vi "test.vi"(8 "COLUMN":i32=9, 9 "ROW":i32=6, 10 "引用":refnum<vi>) -> (0 "料盘ID NG？":bool, 1 "条码1":string[][](array[string]), 2 "条码字符串":string, 3 "托盘ID":string, 4 "工位一NG?":bool, 5 "46~99条码数组":string[](array[string]), 6 "工位1逻辑与":bool)   [LabVIEW 2014]
uses:
  <vilib>/Utility/miscctls.llb/LVRowAndColumnTypeDef.ctl
panel:
  out "已删除的部分 2":string[](array[string])
  out "已删除元素的数组子集 2":string[](array[string])
  out "元素索引 2":i32
  out "数组 3":string[](array[string])
  out "初始化的数组":u32[][](array[numeric])
  out "数组 2":u32[][](array[numeric])
  out "颜色数组":u32[][](array[numeric])
  in  "多列列表框 2":i32[](listbox)
  out "条码数组":string[](array[string])
  out "大小":i32
  out "x-y":dbl
  out "工位1表格":string[][](array[string])
  # "16777238"
  # "Infomation"
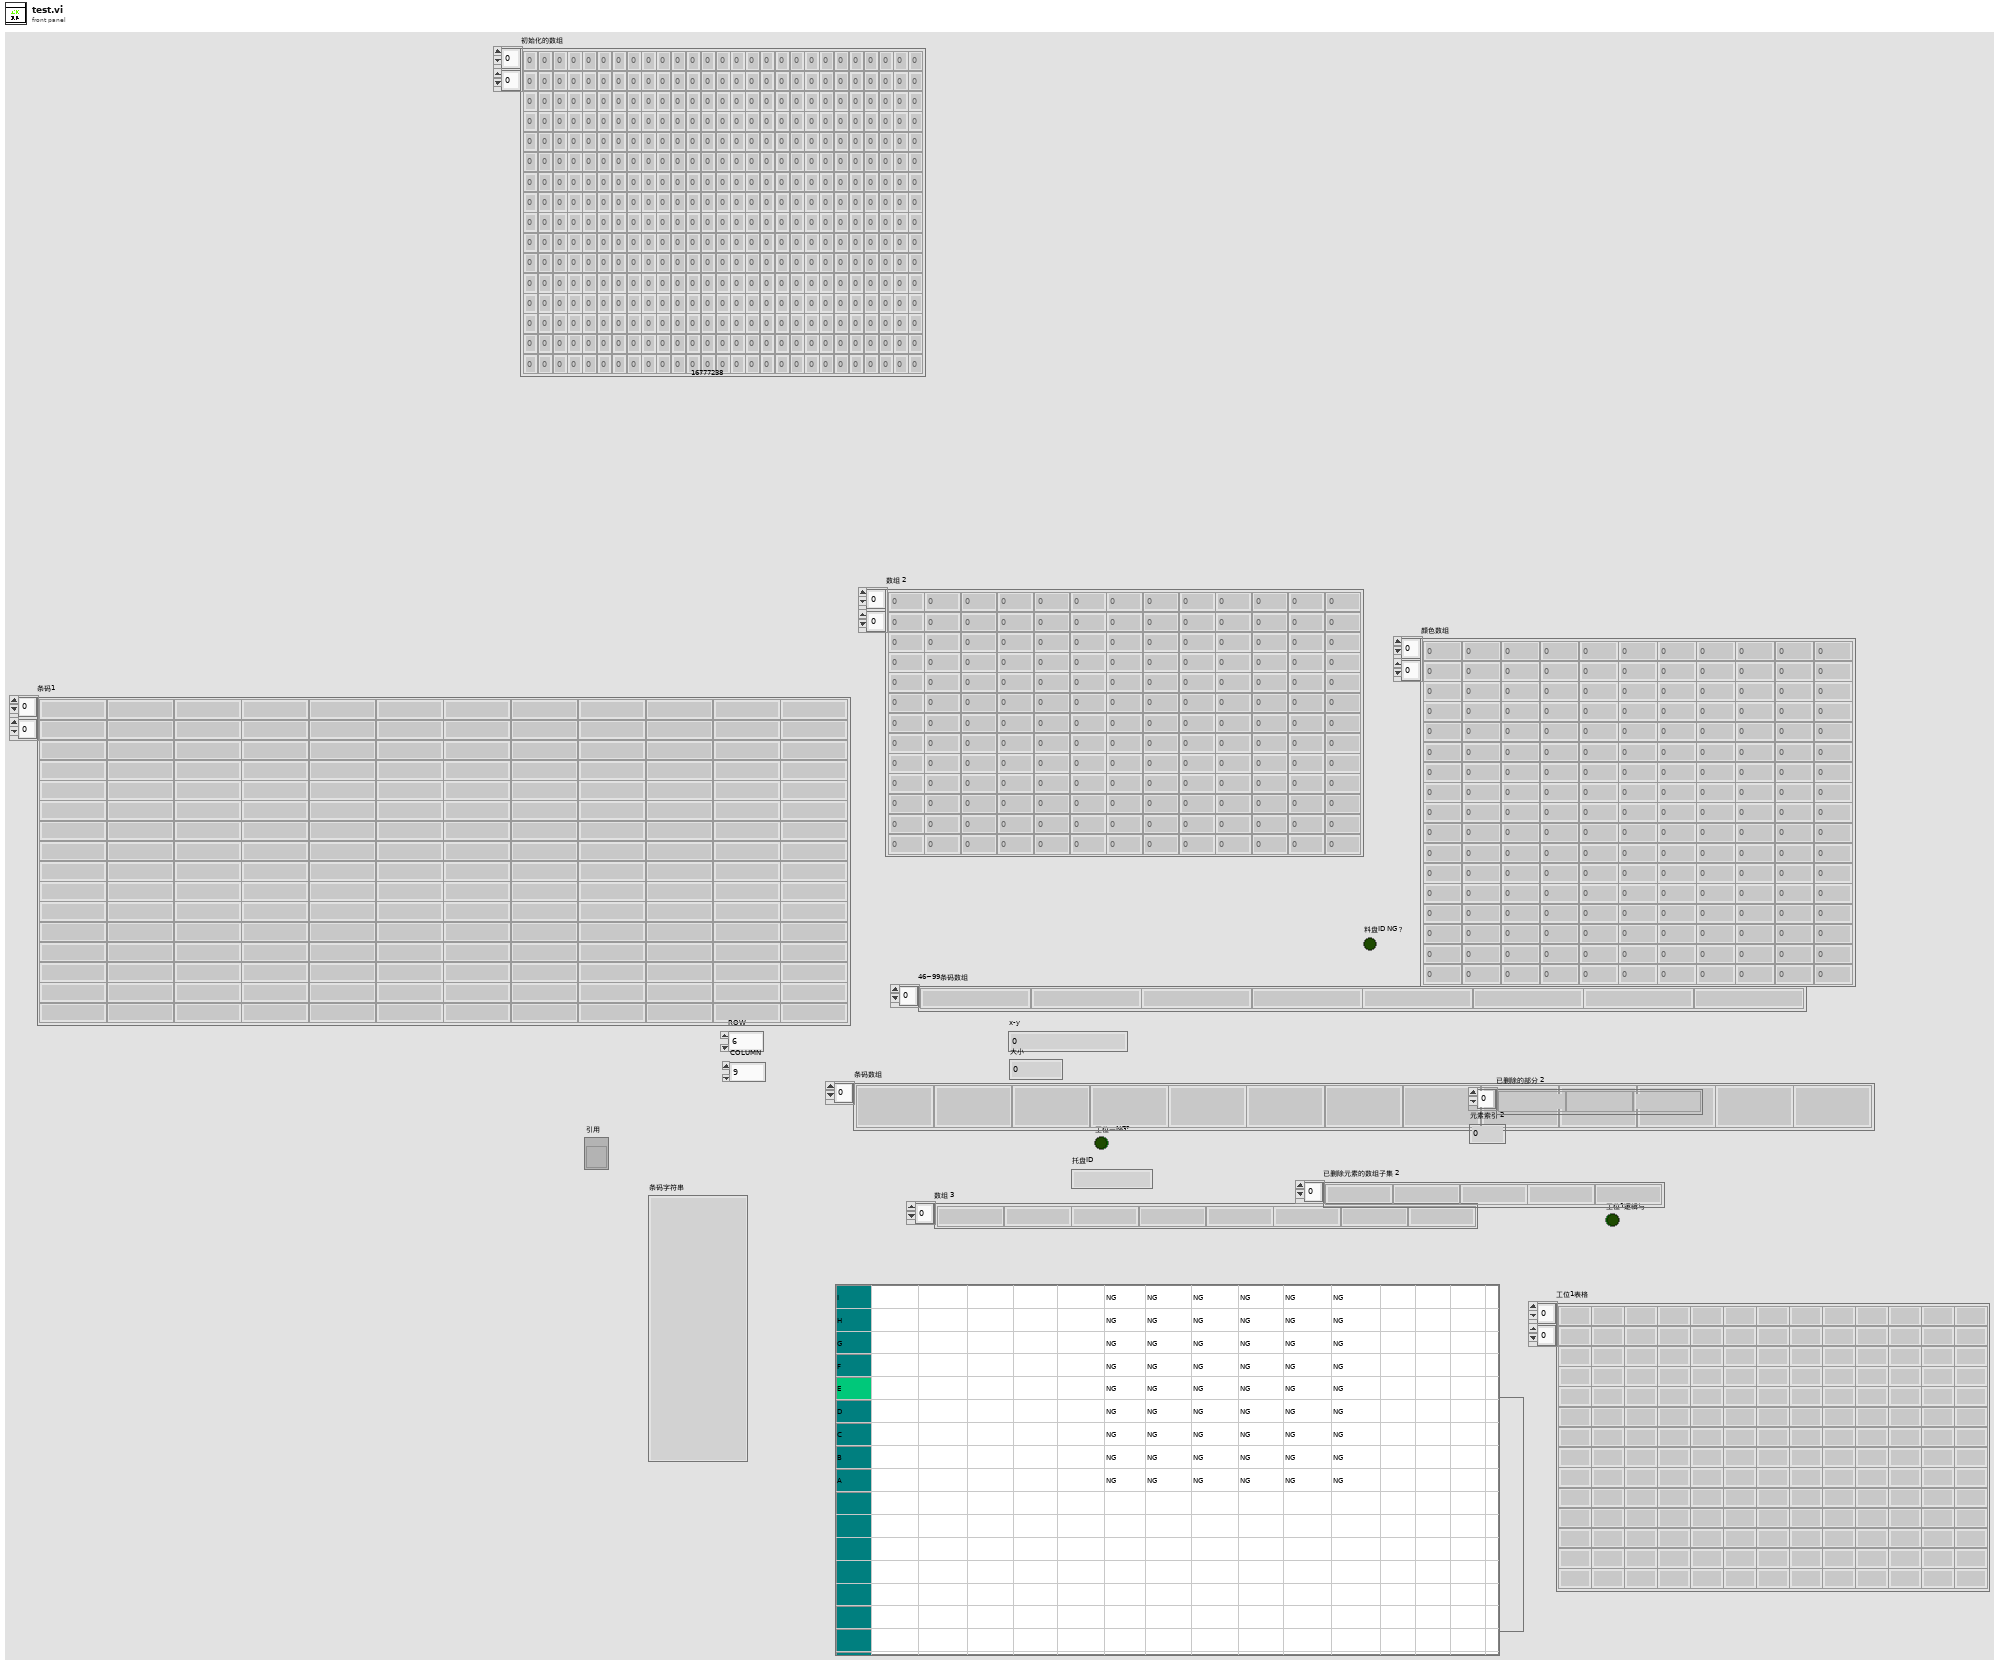
[diagram p1: front panel]
types:
  T1 = typedef "LVRowAndColumnTypeDef.ctl" = cluster{"Row":i32, "Column":i32}
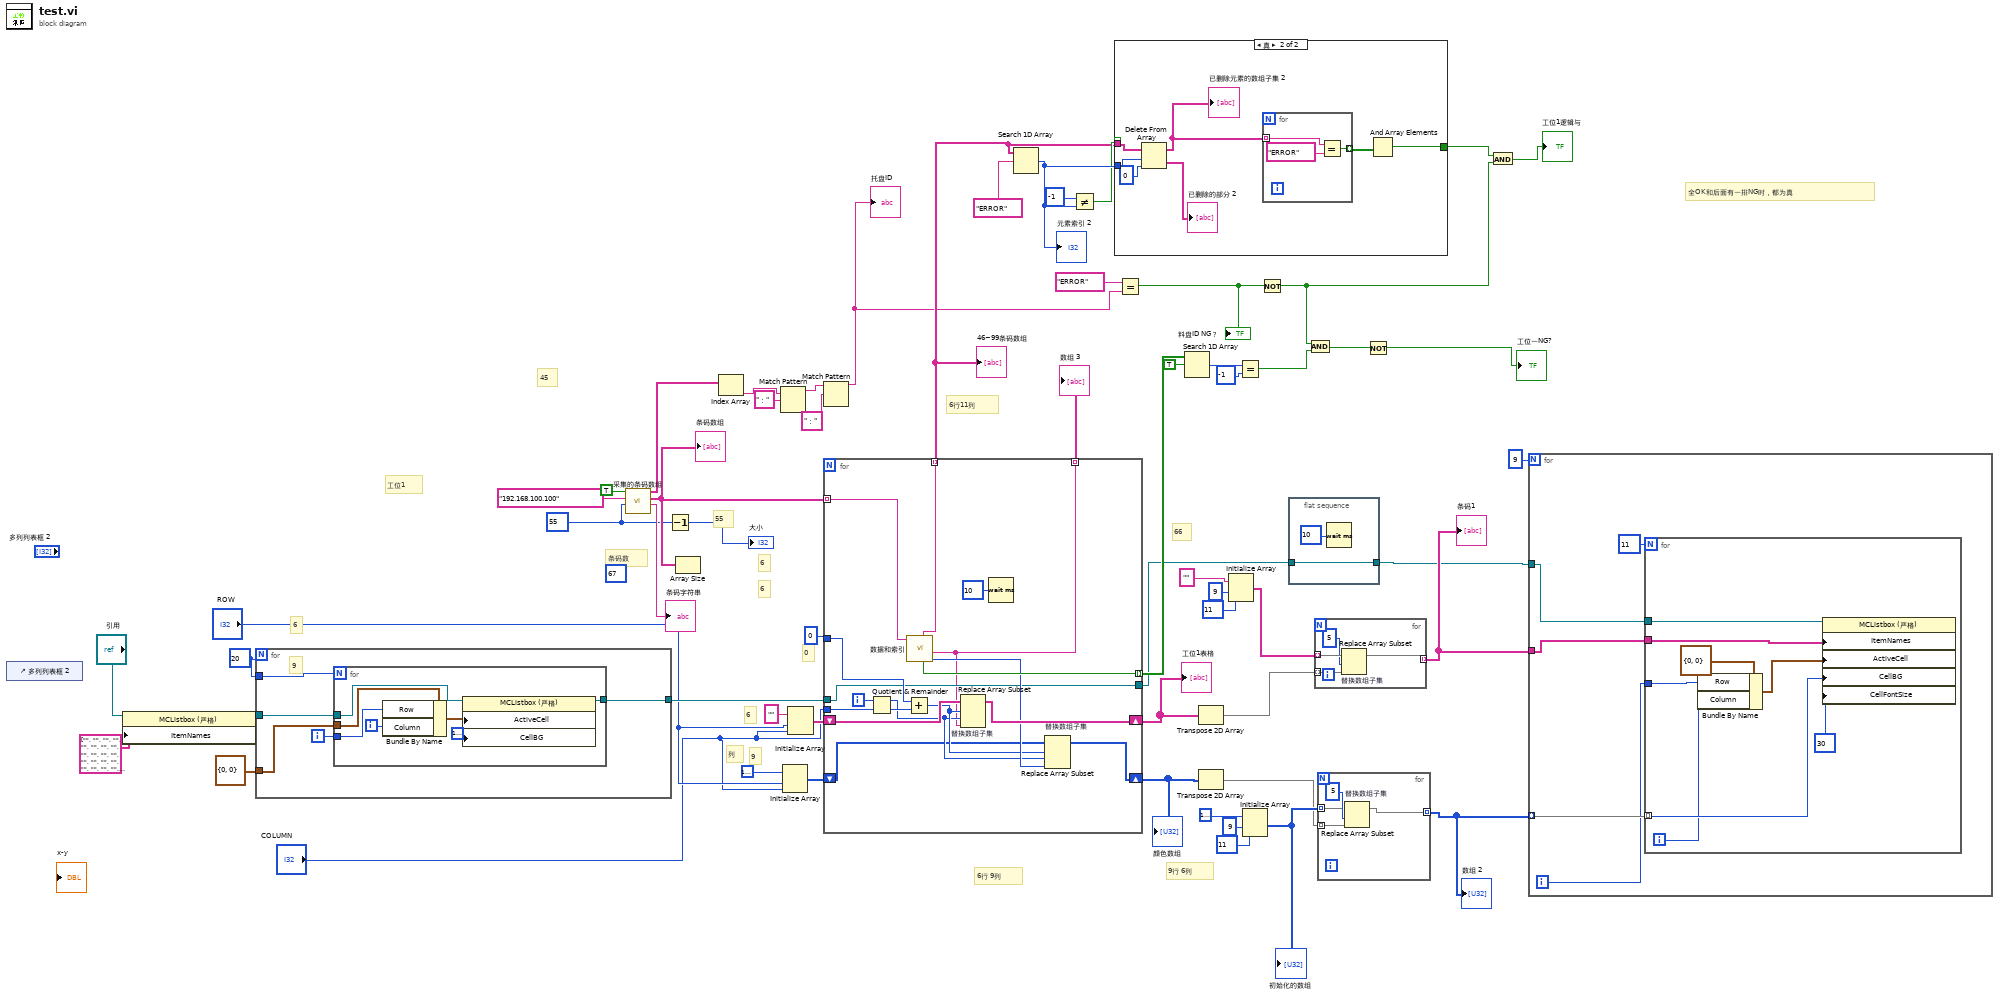
[diagram p0: block diagram]
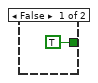
[diagram p2: hidden frame]
diagram:
  w23 = 20
  (unwired) 67
  w46 = 55 ("条码数量")
  # "全OK和后面有一排NG时，都为真"
  # "工位1"
  # "45"
  # "9行 6列"
  # "6行 9列"
  # "66"
  # "6"
  # "6"
  # "6行11列"
  # "0"
  # "条码数"
  # "6"
  # "6"
  # "55"
  # "9"
  # "列"
  n1 = control-ref of="多列列表框 2"() -> ()  [unwired: 1 out]
  n2 = property class="MCListbox (严格)"(reference="引用", "ItemNames"=string[][] [["", "", "", "", "", "", "", "", "", "", ""], ["", "", "", "", "", "", "", "", "", "", ""], ["", "", "", "", "", "", "", "", "", "", ""], ["", "", "", "", "", "", "", "", "", "", ""], ["", "", "", "", "", "", "", "", "", "", ""]] ("项名")) -> (reference out=w58:refnum<vi>)  [unwired: 1 in, 1 out]
  n3 = for {
    N: w23 -> [_]
    tunnel: w58 -> [w65]
    tunnel: T1 {"Row"=0, "Column"=0} ("活动单元格:活动单元格") -> [w64]
    tunnel: [w62] -> w57
    tunnel: w23 -> [w61]
    i -> [w63]
    # "9"
    n4 = for {
      N: w61 -> [_]
      tunnel: w65 -> [w72]
      tunnel: w64 -> [w71]
      tunnel: w63 -> [w69]
      tunnel: [w67] -> w62
      i -> [w68]
      n5 = Bundle By Name(cluster=w71, "Row"=w69, "Column"=w68) -> (w70:T1)
      n6 = property class="MCListbox (严格)"(reference=w72, "ActiveCell"=w70, "CellBG"=u32 16777238) -> (reference out=w67:refnum<vi>)  [unwired: 1 in, 1 out]
    }
  }
  n7 = call "采集的条码数组.vi"("条码数量"=w46, "地址"="192.168.100.100", "开启条码?"=TRUE) -> ("条码字符串"=→"条码字符串":string, "条码数组"=w47:string[], "料号"=w20:string[])  [unwired: 6 in]
  "条码数组" <- w47
  n8 = Decrement(x=w46) -> (x-1=→"大小":i32)
  n9 = Array Size(array=w47) -> ()  [unwired: 1 out]
  n10 = Index Array(array=w20) -> (element=w19:string)  [unwired: 1 in]
  n11 = Match Pattern(string=w19, regular expression="：" ("正则表达式")) -> (before substring=w17:string)  [unwired: 1 in, 3 out]
  n12 = Initialize Array(u32 16777238, "ROW", "COLUMN") -> (w43:u32[][])
  n13 = Initialize Array("", "ROW", "COLUMN") -> (w48:string[][])
  n14 = Match Pattern(string=w17, regular expression="：" ("正则表达式")) -> (before substring=w8:string)  [unwired: 1 in, 3 out]
  "托盘ID" <- w8
  n15 = for {
    tunnel: w47 -> [w89] mode=indexing
    tunnel: w57 -> [w76]
    shift-right: [w88] -> w42
    shift-left: w48 -> [w82]
    tunnel: [w87] -> w56 mode=indexing
    tunnel: "COLUMN" -> [w85]
    tunnel: 0 -> [w83]
    shift-right: [w77] -> w41
    shift-left: w43 -> [w78]
    tunnel: [w76] -> w30
    tunnel: [w74] -> w22 mode=indexing
    tunnel: [w73] -> w10 mode=indexing
    i -> [w86]
    n16 = Quotient & Remainder(x=w86, y=w85) -> (x-y*floor(x/y)=w79:i32, floor(x/y)=w84:i32)
    n17 = Add(x=w83, y=w84) -> (x+y=w80:i32)
    n18 = call "数据和索引.vi"("data out"=w89) -> ("颜色"=w81:u32, "显示数据"=w74:string, "NG?"=w87:bool, "条码"=w73:string)  [unwired: 6 in, 1 out]
    n19 = Replace Array Subset "替换数组子集"(array=w82, new element=w74, index (row)=w80, index (col)=w79) -> (w88:string[][])
    n20 = Wait (ms)(milliseconds to wait=u32 10 ("等待时间（毫秒）")) -> ()  [unwired: 1 out]
    n21 = Replace Array Subset "替换数组子集"(array=w78, new element=w81, index (row)=w80, index (col)=w79) -> (w77:u32[][])
  }
  "工位1表格" <- w42
  "颜色数组" <- w41
  "数组 3" <- w22
  "46~99条码数组" <- w10
  n22 = Search 1D Array(1D array=w10, element="ERROR") -> (index of element=w13:i32)  [unwired: 1 in]
  "元素索引 2" <- w13
  n23 = Not Equal?(x=-1, y=w13) -> (x != y?=w12:bool)
  n24 = case shown="真" w12 {
    tunnel: [TRUE w97] -> w6
    tunnel: w10 -> [_ w96]
    tunnel: w13 -> [_ w95]
    frame False {
    }
    frame True {
      n25 = Delete From Array(array=w96, length=w95, index=0 ("索引")) -> (deleted portion=→"已删除的部分 2":string[], array with subset deleted=w92:string[])
      "已删除元素的数组子集 2" <- w92
      n26 = for {
        tunnel: w92 -> [w100] mode=indexing
        tunnel: [w98] -> w91 mode=indexing
        n27 = Equal?(x=w100, y="ERROR") -> (x = y?=w98:bool)
      }
      n28 = And Array Elements(Boolean array=w91) -> (logical AND=w97:bool)
    }
  }
  n29 = Equal?(x="ERROR", y=w8) -> (x = y?=w7:bool)
  "料盘ID NG？" <- w7
  n30 = Search 1D Array(1D array=w56, element=TRUE) -> (index of element=w54:i32)  [unwired: 1 in]
  n31 = Transpose 2D Array(2D array=w42) -> (transposed array=w35:string[][])
  n32 = Transpose 2D Array(2D array=w41) -> (transposed array=w25:u32[][])
  n33 = Initialize Array("", 9 ("维数大小"), 11 ("维数大小")) -> (w36:string[][])
  n34 = Equal?(x=w54, y=-1) -> (x = y?=w4:bool)
  n35 = Initialize Array(u32 16777238, 9 ("维数大小"), 11 ("维数大小")) -> (w26:u32[][])
  "初始化的数组" <- w26
  n36 = Not(x=w7) -> (.not. x?=w3:bool)
  n37 = flat-sequence {
    tunnel: w30 -> [w102]
    tunnel: [w102] -> w29
    frame #0 {
      n38 = Wait (ms)(milliseconds to wait=u32 10 ("等待时间（毫秒）")) -> ()  [unwired: 1 out]
    }
  }
  n39 = And(x=w3, y=w4) -> (x .and. y?=w2:bool)
  n40 = for {
    tunnel: w36 -> [w106] mode=indexing
    tunnel: w35 -> [w105] mode=indexing
    tunnel: [w103] -> w31 mode=indexing
    n41 = Replace Array Subset "替换数组子集"(array=w106, new element=w105, index=5 ("索引")) -> (w103:string[])
  }
  "条码1" <- w31
  n42 = for {
    tunnel: w26 -> [w107] mode=indexing
    tunnel: w25 -> [w110] mode=indexing
    tunnel: [w108] -> w27 mode=indexing
    n43 = Replace Array Subset "替换数组子集"(array=w107, new element=w110, index=5 ("索引")) -> (w108:u32[])
  }
  "数组 2" <- w27
  n44 = Not(x=w2) -> (.not. x?=→"工位一NG?":bool)
  n45 = And(x=w6, y=w3) -> (x .and. y?=→"工位1逻辑与":bool)
  n46 = for {
    N: 9 -> [_]
    tunnel: w31 -> [w115]
    tunnel: w29 -> [w114]
    tunnel: w27 -> [w113] mode=indexing
    i -> [w111]
    n47 = for {
      N: 11 -> [_]
      tunnel: w115 -> [w123]
      tunnel: w114 -> [w122]
      tunnel: w113 -> [w118] mode=indexing
      tunnel: w111 -> [w117]
      i -> [w116]
      n48 = Bundle By Name(cluster=T1 {"Row"=0, "Column"=0} ("活动单元格:活动单元格"), "Row"=w117, "Column"=w116) -> (w120:T1)
      n49 = property class="MCListbox (严格)"(reference=w122, "ItemNames"=w123, "ActiveCell"=w120, "CellBG"=w118, "CellFontSize"=u32 30 ("活动单元格:单元格字体:字号")) -> ()  [unwired: 1 in, 2 out]
    }
  }
